vi "TwH5DllTest.vi"() -> ()   [LabVIEW 2009]
panel:
  out "XY Graph 3":cluster{"Y":dbl[], "Y":dbl[]}[](graph)
  out "XY Graph 2":cluster{"Y":dbl[], "Y":dbl[]}[](graph)
  out "XY Graph":cluster{"Y":dbl[], "Y":dbl[]}[](graph)
  out "all OK":bool
  out "error out":errorcluster
  in  "error in (no error)":errorcluster
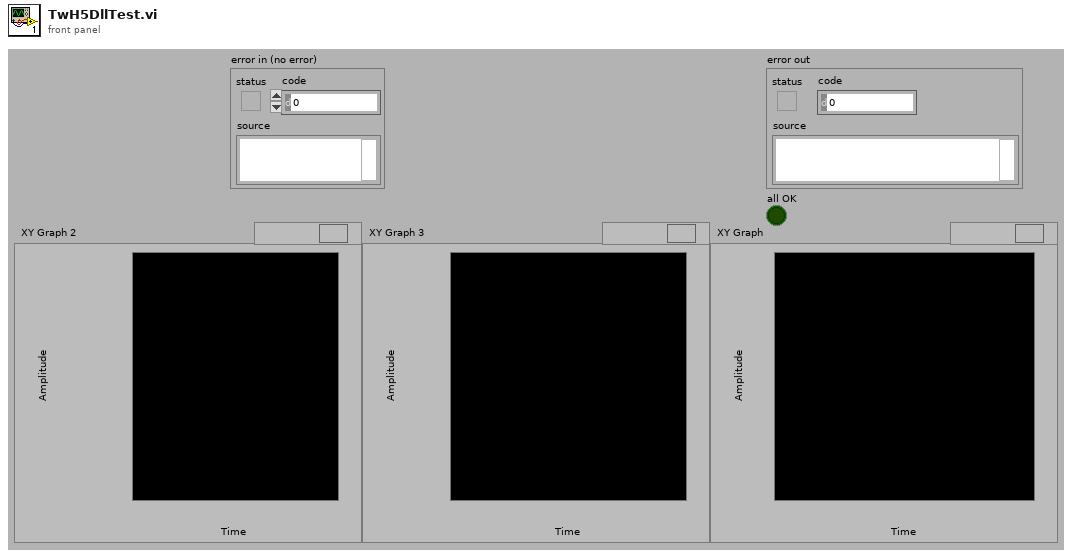
[diagram p1: front panel]
types:
  T1 = cluster{"nbrSamples":i32, "nbrPeaks":i32, "nbrWaveforms":i32, "nbrSegments":i32, "nbrBlocks":i32, "nbrMemories":i32, "nbrBufs":i32, "nbrWrites":i32, "nbrLogEntries":i32, "hasSumSpectrum":u8, "hasBufTimes":u8, "hasTofData":u8, "hasPeakData":u8, "hasTpsData":u8, "hasNbrMemories":u8, "hasPressureData":u8, "hasLogData":u8, "hasMassCalibData":u8, "hasCh1RawData":u8, "hasCh2RawData":u8, "hasRawDataDesc":u8, "daqMode":i32, "acquisitionMode":i32, "massCalibMode":i32, "nbrCalibParams":i32, "p[16]":cluster{"[0]":dbl, "[1]":dbl, "[2]":dbl, "[3]":dbl, "[4]":dbl, "[5]":dbl, "[6]":dbl, "[7]":dbl, "[8]":dbl, "[9]":dbl, "[10]":dbl, "[11]":dbl, "[12]":dbl, "[13]":dbl, "[14]":dbl, "[15]":dbl}, "tofPeriod":dbl, "blockPeriod":dbl, "sampleInterval":sgl, "singleIonSignal":sgl, "dummy5":i32}
  T2 = cluster{"label":string, "mass":sgl, "loMass":sgl, "hiMass":sgl}
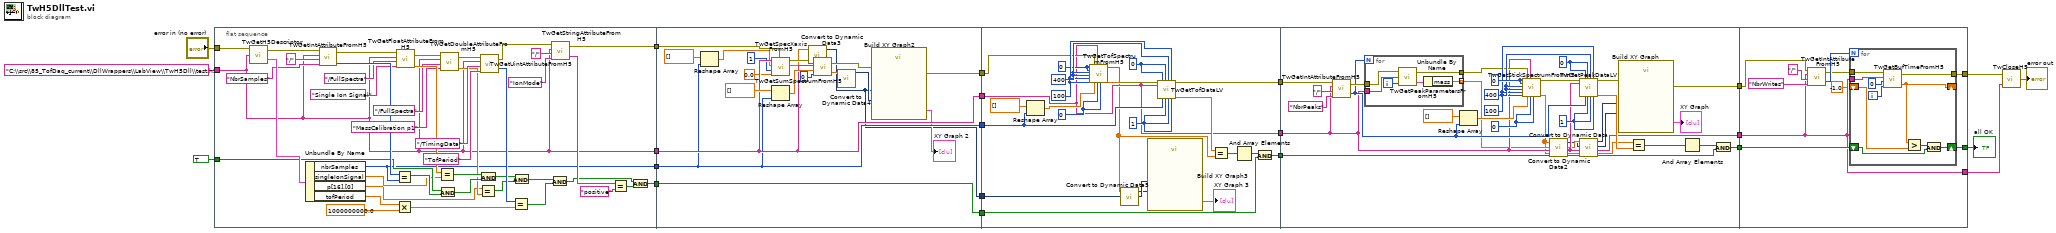
[diagram p0: block diagram]
diagram:
  n1 = flat-sequence {
    tunnel: "C:\\src\\85_TofDaq_current\\DllWrappers\\LabView\\TwH5Dll\\test.h5" ("filename") -> [w24]
    tunnel: "error in (no error)" -> [w63]
    tunnel: TRUE -> [w57]
    tunnel: [w26] -> w19
    tunnel: [w25] -> w18
    tunnel: [w24] -> w17
    tunnel: [w23] -> w16
    tunnel: w19 -> [w78]
    tunnel: w18 -> [w83]
    tunnel: w17 -> [w79]
    tunnel: w16 -> [w72]
    tunnel: [w83] -> w15
    tunnel: [w66] -> w14
    tunnel: [w79] -> w13
    tunnel: [w72] -> w12
    tunnel: [w65] -> w4
    tunnel: w15 -> [w94]
    tunnel: w14 -> [w92]
    tunnel: w13 -> [w90]
    tunnel: w12 -> [w91]
    tunnel: [w90] -> w9
    tunnel: [w89] -> w8
    tunnel: [w88] -> w7
    tunnel: w4 -> [w86]
    tunnel: w9 -> [w113]
    tunnel: w8 -> [w132]
    tunnel: w7 -> [w125]
    tunnel: [w113] -> w3
    tunnel: [w118] -> w2
    tunnel: [w106] -> w1
    tunnel: [w144] -> w5
    tunnel: [w142] -> w6
    tunnel: [w141] -> w11
    tunnel: w3 -> [w141]
    tunnel: w2 -> [w143]
    tunnel: w1 -> [w147]
    frame #0 {
      n2 = call "TwGetH5Descriptor.vi"("filename"=w24, "error in (no error)"=w63) -> ("TwH5Desc out"=w64:T1, "error out"=w62:errorcluster)  [unwired: 1 in]
      n3 = Unbundle By Name(w64) -> ("nbrSamples"=w23:i32, "singleIonSignal"=w53:sgl, "p[16].[0]"=w37:dbl, "tofPeriod"=w47:dbl)
      n4 = call "TwGetIntAttributeFromH5.vi"("name"="NbrSamples", "location"="/", "filename"=w24, "error in (no error)"=w62) -> ("attribute"=w59:i32, "error out"=w54:errorcluster)
      n5 = Equal?(x=w59, y=w23) -> (x = y?=w58:bool)
      n6 = Multiply(x=w47, y=1000000000.0) -> (x*y=w44:dbl)
      n7 = call "TwGetFloatAttributeFromH5.vi"("name"="Single Ion Signal", "location"="/FullSpectra", "filename"=w24, "error in (no error)"=w54) -> ("attribute"=w52:sgl, "error out"=w42:errorcluster)
      n8 = Equal?(x=w52, y=w53) -> (x = y?=w50:bool)
      n9 = And(x=w57, y=w58) -> (x .and. y?=w51:bool)
      n10 = call "TwGetDoubleAttributeFromH5.vi"("name"="MassCalibration p1", "location"="/FullSpectra", "filename"=w24, "error in (no error)"=w42) -> ("attribute"=w38:dbl, "error out"=w41:errorcluster)
      n11 = Equal?(x=w37, y=w38) -> (x = y?=w31:bool)
      n12 = And(x=w50, y=w51) -> (x .and. y?=w36:bool)
      n13 = call "TwGetUintAttributeFromH5.vi"("name"="TofPeriod", "location"="/TimingData", "filename"=w24, "error in (no error)"=w41) -> ("attribute"=w45:u32, "error out"=w34:errorcluster)
      n14 = Equal?(x=w45, y=w44) -> (x = y?=w43:bool)
      n15 = And(x=w36, y=w31) -> (x .and. y?=w35:bool)
      n16 = And(x=w35, y=w43) -> (x .and. y?=w27:bool)
      n17 = call "TwGetStringAttributeFromH5.vi"("name"="IonMode", "location"="/", "filename"=w24, "error in (no error)"=w34) -> ("attribute"=w30:string, "error out"=w26:errorcluster)
      n18 = Equal?(x=w30, y="positive" ("x")) -> (x = y?=w28:bool)
      n19 = And(x=w27, y=w28) -> (x .and. y?=w25:bool)
    }
    frame #1 {
      n20 = Reshape Array(dbl[] [] ("array"), w72) -> (w73:dbl[])
      n21 = call "TwGetSpecXaxisFromH5.vi"("error in (no error)"=w78, "maxMass"=0.0, "axisType"=1, "specAxis in"=w73, "filename"=w79) -> ("specAxis out"=w70:dbl[], "error out"=w77:errorcluster)  [unwired: 2 in, 1 out]
      n22 = Reshape Array(dbl[] [] ("array"), w72) -> (w80:dbl[])
      n23 = call "Convert to Dynamic Data3"("Array"=w70) -> ("Dynamic Data Type"=w65:dynamicdata)  [unwired: 3 in]
      n24 = call "TwGetSumSpectrumFromH5.vi"("normalize"=u8 0, "spectrum in"=w80, "filename"=w79, "error in (no error)"=w77) -> ("spectrum out"=w69:dbl[], "error out"=w67:errorcluster)
      n25 = call "Convert to Dynamic Data4"("Array"=w69) -> ("Dynamic Data Type"=w68:dynamicdata)  [unwired: 3 in]
      n26 = call "Build XY Graph2"("error in (no error)"=w67, "Y Input"=w68, "X Input"=w65) -> ("error out"=w66:errorcluster, "XY Graph"=→"XY Graph 2":cluster{"Y":dbl[], "Y":dbl[]}[])  [unwired: 7 in]
    }
    frame #2 {
      w100 = 0 ("sampleOffset")
      w101 = 1 ("segCount")
      w98 = 100 ("writeIndex")
      w99 = 400 ("bufIndex")
      w93 = 0 ("segmentIndex")
      w103 = u8 0 ("bufWriteLinked")
      n27 = Reshape Array(sgl[] [] ("array"), w91) -> (w105:sgl[])
      n28 = call "TwGetTofSpectrumFromH5.vi"("segmentIndex"=w93, "segmentEndIndex"=w93, "bufIndex"=w99, "bufEndIndex"=w99, "writeIndex"=w98, "writeEndIndex"=w98, "error in (no error)"=w92, "spectrum in"=w105, "filename"=w90, "bufWriteLinked"=w103, "normalize"=w103) -> ("error out"=w102:errorcluster, "spectrum out"=w85:sgl[])  [unwired: 7 in]
      n29 = call "Convert to Dynamic Data5"("Array"=w85) -> ("Dynamic Data Type"=w84:dynamicdata)  [unwired: 3 in]
      n30 = call "Build XY Graph3"("Y Input"=w84, "X Input"=w86) -> ("XY Graph"=→"XY Graph 3":cluster{"Y":dbl[], "Y":dbl[]}[])  [unwired: 8 in, 1 out]
      n31 = call "TwGetTofDataLV.vi"("error in (no error)"=w102, "filename"=w90, "sampleOffset"=w100, "sampleCount"=w91, "segOffset"=w100, "segCount"=w101, "bufOffset"=w99, "bufCount"=w101, "writeOffset"=w98, "writeCount"=w101) -> ("error out"=w89:errorcluster, "dataBuffer"=w97:sgl[])  [unwired: 8 in]
      n32 = Equal?(x=w97, y=w85) -> (x = y?=w96:bool[])
      n33 = And Array Elements(Boolean array=w96) -> (logical AND=w95:bool)
      n34 = And(x=w95, y=w94) -> (x .and. y?=w88:bool)
    }
    frame #3 {
      w119 = 100 ("writeIndex")
      w120 = 400 ("bufIndex")
      w121 = 0 ("peakOffset")
      w122 = 0 ("segmentIndex")
      w123 = 1 ("segCount")
      w124 = u8 0 ("bufWriteLinked")
      n35 = call "TwGetIntAttributeFromH5.vi"("name"="NbrPeaks", "location"="/", "filename"=w113, "error in (no error)"=w132) -> ("attribute"=w115:i32, "error out"=w117:errorcluster)
      n36 = for {
        N: w115 -> [_]
        tunnel: w117 -> [w139]
        tunnel: [w138] -> w116
        tunnel: [w135] -> w111 mode=indexing
        tunnel: w113 -> [w134]
        i -> [w137]
        n37 = call "TwGetPeakParametersFromH5.vi"("PeakIndex"=w137, "filename"=w134, "error in (no error)"=w139) -> ("PeakPar out"=w136:T2, "error out"=w138:errorcluster)
        n38 = Unbundle By Name(w136) -> ("mass"=w135:sgl)
      }
      n39 = Reshape Array(sgl[] [] ("array"), w115) -> (w128:sgl[])
      n40 = call "TwGetStickSpectrumFromH5.vi"("segmentIndex"=w122, "segmentEndIndex"=w122, "bufIndex"=w120, "bufEndIndex"=w120, "writeIndex"=w119, "writeEndIndex"=w119, "error in (no error)"=w116, "spectrum in"=w128, "filename"=w113, "bufWriteLinked"=w124, "normalize"=w124) -> ("error out"=w133:errorcluster, "spectrum out"=w109:sgl[])  [unwired: 7 in]
      n41 = call "Convert to Dynamic Data2"("Array"=w109) -> ("Dynamic Data Type"=w108:dynamicdata)  [unwired: 3 in]
      n42 = call "TwGetPeakDataLV.vi"("error in (no error)"=w133, "filename"=w113, "peakOffset"=w121, "peakCount"=w115, "segOffset"=w121, "segCount"=w123, "bufOffset"=w120, "bufCount"=w123, "writeOffset"=w119, "writeCount"=w123) -> ("error out"=w107:errorcluster, "dataBuffer"=w114:sgl[])  [unwired: 8 in]
      n43 = call "Convert to Dynamic Data"("Array"=w111) -> ("Dynamic Data Type"=w110:dynamicdata)  [unwired: 3 in]
      n44 = call "Build XY Graph"("error in (no error)"=w107, "Y Input"=w108, "X Input"=w110) -> ("error out"=w106:errorcluster, "XY Graph"=→"XY Graph":cluster{"Y":dbl[], "Y":dbl[]}[])  [unwired: 7 in]
      n45 = Equal?(x=w109, y=w114) -> (x = y?=w127:bool[])
      n46 = And Array Elements(Boolean array=w127) -> (logical AND=w126:bool)
      n47 = And(x=w126, y=w125) -> (x .and. y?=w118:bool)
    }
    frame #4 {
      n48 = call "TwGetIntAttributeFromH5.vi"("name"="NbrWrites", "location"="/", "filename"=w141, "error in (no error)"=w147) -> ("attribute"=w146:i32, "error out"=w145:errorcluster)
      n49 = for {
        N: w146 -> [_]
        tunnel: w145 -> [w157]
        tunnel: [w156] -> w144
        shift-right: [w155] -> _
        shift-left: -1.0 ("bufTime") -> [w154]
        shift-right: [w152] -> w142
        shift-left: w143 -> [w151]
        tunnel: w141 -> [w150]
        i -> [w159]
        n50 = call "TwGetBufTimeFromH5.vi"("writeIndex"=w159, "bufIndex"=0, "filename"=w150, "error in (no error)"=w157) -> ("bufTime"=w155:dbl, "error out"=w156:errorcluster)
        n51 = Greater?(x=w155, y=w154) -> (0:w153:bool)
        n52 = And(x=w153, y=w151) -> (x .and. y?=w152:bool)
      }
    }
  }
  n53 = call "TwCloseH5.vi"("filename"=w11, "error in (no error)"=w5) -> ("error out"=→"error out":errorcluster)
  "all OK" <- w6
